vi "KH7008 COM.vi"(8 "error in (no error)":errorcluster, 10 "Command":string, 11 "VISA Refnum in":refnum<visa-resource-name>="COM3") -> (0 "error out":errorcluster, 2 "Response":string="\r\n")   [LabVIEW 2016, in "Instrument.KH7008.lvclass"]
uses:
  Instrument.KH7008.lvclass
  <vilib>/Instr/_visa.llb/VISA Configure Serial Port (Instr).vi
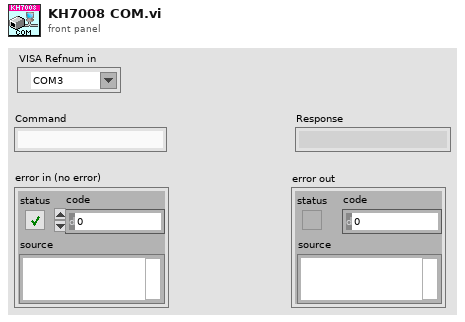
[diagram p1: front panel]
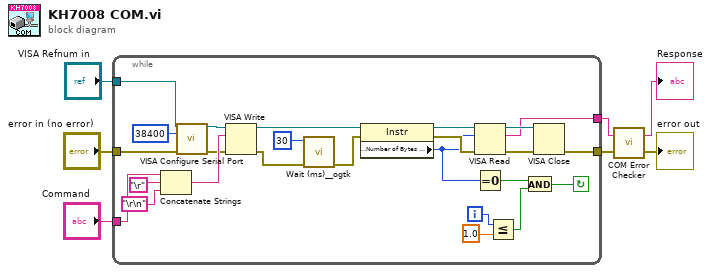
[diagram p0: block diagram]
diagram:
  n1 = while {
    tunnel: "VISA Refnum in" -> [w20]
    tunnel: "Command" -> [w19]
    tunnel: "error in (no error)" -> [w13]
    tunnel: [w12] -> w4
    tunnel: [w11] -> w1
    i -> [w17]
    stop <- w14 continue-if-true
    n2 = Concatenate Strings(w19, "\r", "\r\n") -> (w32:string)
    n3 = call-poly "VISA Configure Serial Port"("VISA resource name"=w20, "baud rate (9600)"=u32 38400 ("baud rate"), "error in (no error)"=w13) -> ("VISA resource name out"=w28:refnum<visa-resource-name>, "error out"=w29:errorcluster)  [unwired: 6 in, 5 out]
    n4 = VISA Write(VISA resource name=w28, write buffer=w32, error in (no error)=w29) -> (VISA resource name out=w25:refnum<visa-resource-name>, error out=w24:errorcluster)  [unwired: 1 out]
    n5 = call <userlib>:"Wait (ms)__ogtk.vi"("error in (no error)"=w24, "milliseconds to wait"=u32 30) -> ("error out"=w9:errorcluster)  [unwired: 8 in, 1 out]
    n6 = property class="Instr"(reference=w25, error in=w9) -> (reference out=w26:refnum<visa-resource-name>, error out=w27:errorcluster, "Serial Settings:Number of Bytes at Serial Port"=w8:u32)
    n7 = VISA Read(VISA resource name=w26, byte count=w8, error in (no error)=w27) -> (VISA resource name out=w23:refnum<visa-resource-name>, read buffer=w11:string, error out=w22:errorcluster)  [unwired: 1 out]
    n8 = Equal To 0?(x=w8) -> (x = 0?=w16:bool)
    n9 = Less Or Equal?(x=w17, y=1.0) -> (x <= y?=w15:bool)
    n10 = And(x=w16, y=w15) -> (x .and. y?=w14:bool)
    n11 = VISA Close(VISA resource name=w23, error in (no error)=w22) -> (error out=w12:errorcluster)
  }
  n12 = call "COM Error Checker.vi"("error in (no error)"=w4, "String In"=w1) -> ("error out"=→"error out":errorcluster, "String"=→"Response":string)
